vi "svx_Orbit and Timebase Segment (Unfiltered).vi"(5 "reset? (F)":bool, 6 "end reach?":bool, 8 "error in (no error)":errorcluster, 9 "indice":cluster{"start":i32, "length":i32}, 11 "resampled signal in":cluster{"r0":dbl, "dr":dbl, "Y":dbl[]}[](array[cluster]) {"r0" format="%.2p"; "dr" format="%.2p"; "Y" format="%.2f"}) -> (0 "error out":errorcluster, 3 "resampled signal out":cluster{dbl[], dbl}[](array[cluster]))   [LabVIEW 2017]
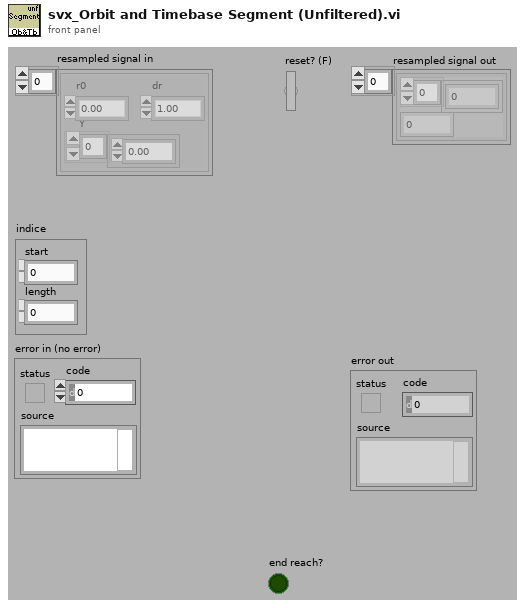
[diagram p1: front panel]
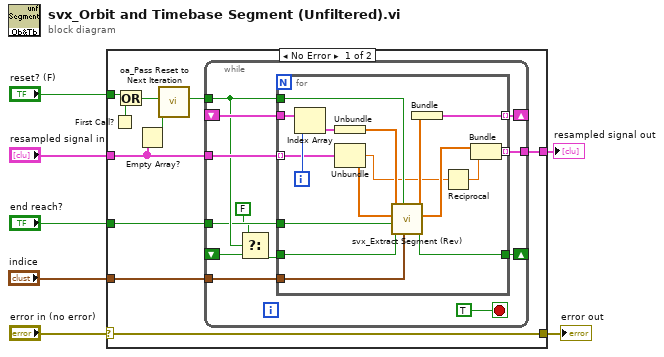
[diagram p0: block diagram]
diagram:
  n1 = case shown="No Error" "error in (no error)" {
    selector: "error in (no error)" -> [w15 w47]
    tunnel: "reset? (F)" -> [w17 _]
    tunnel: "resampled signal in" -> [w13 _]
    tunnel: [w15 w47] -> w4
    tunnel: "end reach?" -> [w10 _]
    tunnel: "indice" -> [w9 _]
    tunnel: [w8 _] -> w2
    frame No Error {
      n2 = First Call?() -> (First Call?: T/F=w16:bool)
      n3 = Or(x=w17, y=w16) -> (x .or. y?=w12:bool)
      n4 = Empty Array?(array=w13) -> (empty?=w14:bool)
      n5 = call <vilib>:"oa_Pass Reset to Next Iteration.vi"("trigger"=w14, "reset?(F)"=w12) -> ("reset out"=w11:bool)  [unwired: 9 in]
      n6 = while {
        tunnel: w13 -> [w28]
        shift-right: [w23] -> _
        shift-left: _ -> [w27]
        tunnel: w11 -> [w22]
        shift-right: [w25] -> _
        shift-left: _ -> [w21]
        tunnel: [w24] -> w8
        tunnel: w10 -> [w20]
        tunnel: w9 -> [w26]
        stop <- TRUE stop-if-true
        n7 = Select(t=FALSE, s=w22, f=w21) -> (s? t:f=w19:bool)
        n8 = for {
          tunnel: w28 -> [w44] mode=indexing
          tunnel: w27 -> [w46]
          tunnel: w22 -> [w42]
          tunnel: w19 -> [w38]
          tunnel: [w33] -> w24 mode=indexing
          tunnel: w20 -> [w39]
          tunnel: w26 -> [w30]
          tunnel: [w37] -> w25
          tunnel: [w35] -> w23 mode=indexing
          i -> [w45]
          n9 = Index Array(array=w46, index=w45) -> (element=w43:cluster{"remaining data ":dbl[]})
          n10 = Unbundle(w43) -> ("remaining data"=w41:dbl[])
          n11 = Unbundle(w44) -> ("dr"=w32:dbl, "Y"=w40:dbl[])  [unwired: 1 out]
          n12 = call <vilib>:"svx_Extract Segment (Rev).vi"("indice"=w30, "reset?"=w42, "old end reached"=w38, "end reached"=w39, "data in"=w40, "old order data"=w41) -> ("end reached out"=w37:bool, "data out"=w34:dbl[], "remaining data"=w36:dbl[])  [unwired: 3 in]
          n13 = Bundle("remaining data"=w36) -> (w35:cluster{"remaining data ":dbl[]})  [unwired: 1 in]
          n14 = Reciprocal(x=w32) -> (1/x=w31:dbl)
          n15 = Bundle("data out"=w34, w31) -> (w33:cluster{"data out":dbl[], dbl})  [unwired: 1 in]
        }
      }
    }
    frame Error {
    }
  }
  "resampled signal out" <- w2
  "error out" <- w4
